vi "dfd_Get Total Height_Width.vi"(11 "Array":cluster{"Width":u32, "Height":u32}[](array[cluster])) -> (3 "Bounds":cluster{"Width":u32, "Height":u32})   [LabVIEW 2017, in "NI_DigFilter_Process.lvlib"]
uses:
  <vilib>/addons/Digital Filter Design/NI_DigFilter_Process.lvlib
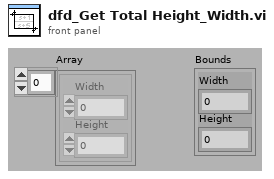
[diagram p1: front panel]
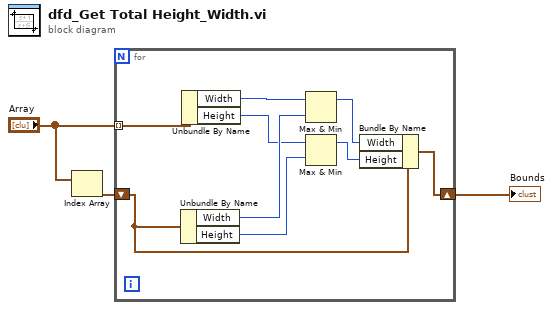
[diagram p0: block diagram]
diagram:
  n1 = Index Array(array="Array") -> (element=w3:cluster{"Width":u32, "Height":u32})  [unwired: 1 in]
  n2 = for {
    shift-right: [w8] -> w1
    shift-left: w3 -> [w4]
    tunnel: "Array" -> [w9] mode=indexing
    n3 = Unbundle By Name(w4) -> ("Width"=w11:u32, "Height"=w12:u32)
    n4 = Unbundle By Name(w9) -> ("Width"=w7:u32, "Height"=w10:u32)
    n5 = Max & Min(x=w7, y=w11) -> (max(x,y)=w6:u32)  [unwired: 1 out]
    n6 = Max & Min(x=w10, y=w12) -> (max(x,y)=w5:u32)  [unwired: 1 out]
    n7 = Bundle By Name(cluster=w4, "Width"=w6, "Height"=w5) -> (w8:cluster{"Width":u32, "Height":u32})
  }
  "Bounds" <- w1
